vi "Construct.vi"(8 "error in (no error)":errorcluster, 10 "Initital memory allocation":i32=1024, 11 "Outline in":refnum<class "Outline.lvclass">) -> (0 "error out":errorcluster, 3 "Outline out":refnum<class "Outline.lvclass">)   [LabVIEW 2013, in "Outline.lvclass"]
uses:
  Outline.lvclass
  Outline.lvclass/Outline.ctl
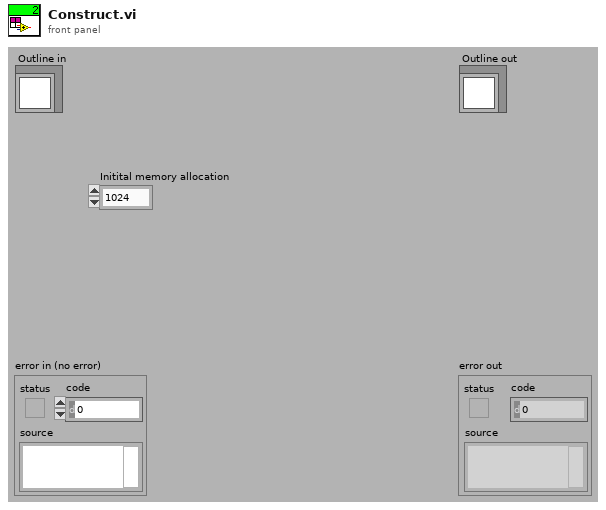
[diagram p1: front panel]
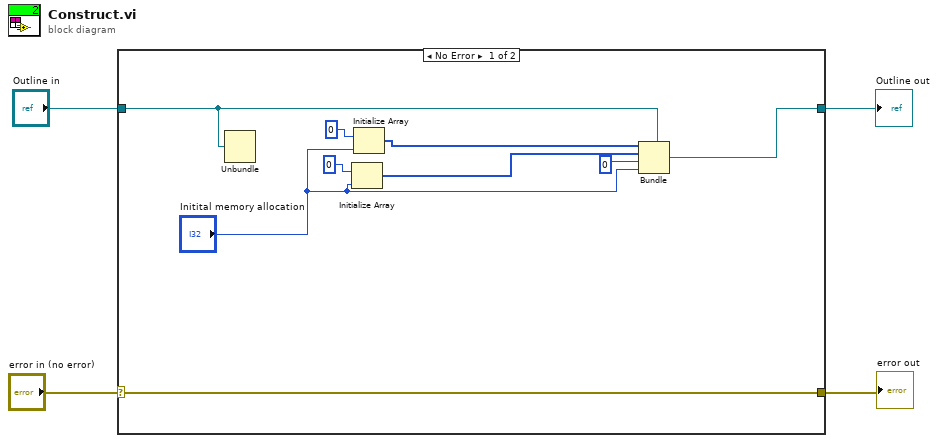
[diagram p0: block diagram]
diagram:
  n1 = case shown="No Error" "error in (no error)" {
    selector: "error in (no error)" -> [w13 w15]
    tunnel: [w13 w15] -> w3
    tunnel: [w11 w14] -> w1
    tunnel: "Outline in" -> [w12 w14]
    frame No Error {
      n2 = Unbundle(w12) -> ()  [unwired: 4 out]
      n3 = Initialize Array(0, "Initital memory allocation") -> (w6:i32[])
      n4 = Initialize Array(0, "Initital memory allocation") -> (w8:i32[])
      n5 = Bundle(cluster=w12, w8, w6, 0 ("Number of points"), "Initital memory allocation") -> (w11:refnum<class "Outline.lvclass">)
    }
    frame Error {
    }
  }
  "error out" <- w3
  "Outline out" <- w1
